vi "Write Offset Measured.vi"(10 "Offset Measured":dbl[unit] format="%.1f", 11 "ForceSensor in":refnum<class "ForceSensor.lvclass">) -> (3 "ForceSensor out":refnum<class "ForceSensor.lvclass">)   [LabVIEW 2013, in "ForceSensor.lvclass"]
uses:
  ForceSensor.lvclass
  ForceSensor.lvclass/ForceSensor.ctl
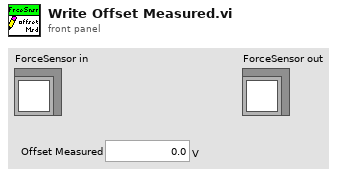
[diagram p1: front panel]
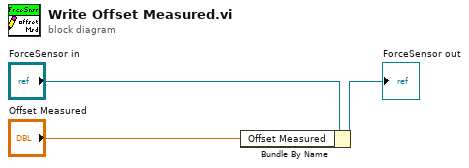
[diagram p0: block diagram]
diagram:
  n1 = Bundle By Name(cluster="ForceSensor in", "Offset Measured"="Offset Measured") -> (→"ForceSensor out":refnum<class "ForceSensor.lvclass">)
